vi "_STP.vi"(0 "System no.":i32=1 min=1 max=4 step=1, 2 "Affected axes?":string[](array[string]), 3 "All axes?":bool, 4 "Axis identifier?":bool=TRUE, 5 "error in":errorcluster) -> (19 "error out":errorcluster)   [LabVIEW 2018]
doc: "Stops motion of specified axes. To stop a referencing routine (REF, MNL, MPL) or fast scan routine (FSC, FSA etc.), or AutoZero procedure (ATZ), or wave generator run (WGO), use \"#24.vi\". STP sets error code 10, call \"ERR?.vi\" to reset error after STP has been called.\n\nValid for Analog systems, C-702, C-843, C-843.PM, C-844, C-848, C-865, C-866, C-867, C-880, E-516, E-517, E-712, E-725, E-753, E755, E-761, E-861, Mercury™ (but must be present for E-710 also). To support analog interfacing, VI must be present for E-816 also.\n\nAnalog: All axes = TRUE, Axis identifier = FALSE. STP does not set any error code.\nC-702: All axes = TRUE, Axis identifier = FALSE\nC-843: All axes = TRUE, Axis identifier = FALSE\nC-843.PM: All axes = TRUE, Axis identifier = FALSE\nC-844: All axes = TRUE, Axis identifier = FALSE\nC-848: All axes = TRUE, Axis identifier = FALSE\nC-865: All axes = TRUE, Axis identifier = FALSE\nC-866: All axes = TRUE, Axis identifier = FALSE\nC-867: All axes? = TRUE, Axis identifier? = FALSE\nC-880: All axes = TRUE, Axis identifier = FALSE \nE-516: If All axes = TRUE, then Axis identifier must be TRUE\nE-517: All axes? = TRUE, Axis identifier? = FALSE. STP.vi stops motion of all axes caused by move commands (MOV, MVR, GOH, SVA, SVR). Furthermore, it stops macros (MAC) and wave generator output (WGO).\nE-712, E-725, E-753: If All axes? = TRUE, then Axis identifier? can be FALSE. STP.vi stops motion of all axes caused by move commands (MOV, MVR, SVA, SVR), by the wave generator (WGO), by analog control input and autozero motion (ATZ).\nE-755: If All axes? = TRUE, then Axis identifier can be FALSE\nE-761: All axes = TRUE, Axis identifier = FALSE\nE-861: All axes? = TRUE, Axis identifier? = FALSE\nMercury: All axes = TRUE, Axis identifier = FALSE"
panel:
  # "Stops the motion of the specified axes.\n(To stop a referencing routine or firmware internal\nfast scan routines, or AutoZero procedure, or wave\ngenerator run, use \"#24.vi\")"
  # "If all axes: use"
  # "Stop"
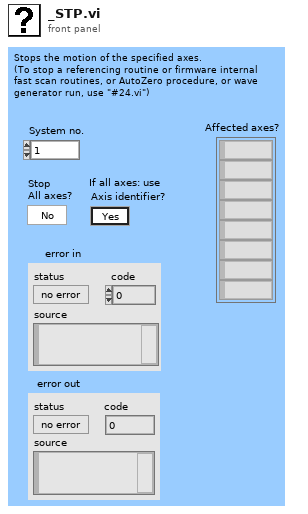
[diagram p1: front panel]
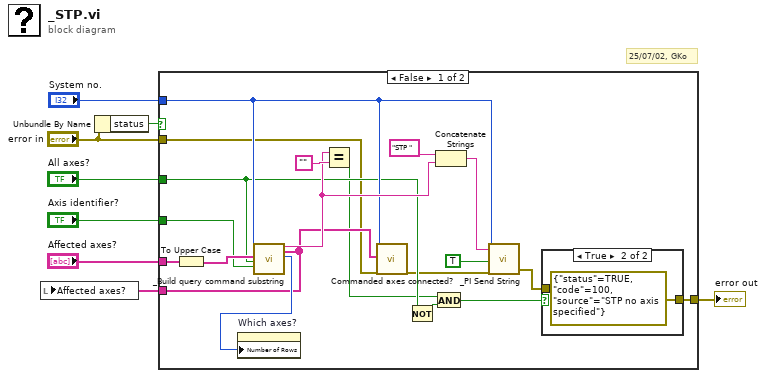
[diagram p0: block diagram]
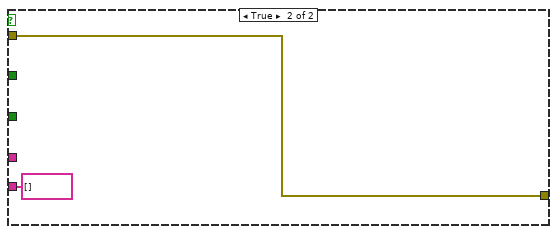
[diagram p3: hidden frame]
diagram:
  # "25/07/02, GKo"
  n1 = Unbundle By Name("error in") -> ("status"=w1:bool)
  n2 = case shown="False" w1 {
    tunnel: "Affected axes?" -> [w24 _]
    tunnel: [w21 w30] -> w7
    tunnel: "Axis identifier?" -> [w19 _]
    tunnel: "System no." -> [w16 _]
    tunnel: [w15 string[] [] ("Axes to query out")] -> w4
    tunnel: "All axes?" -> [w14 _]
    tunnel: "error in" -> [w9 w30]
    frame False {
      n3 = To Upper Case(1:w24) -> (0:w20:string[])
      n4 = call "_Build query command substring.vi"("System no."=w16, "Axes to query in"=w20, "Query\nAll axes?"=w14, "For all axes: use\nAxis identifier?"=w19) -> ("Command substring"=w18:string, "Axes to query out"=w15:string[], "Number of rows"=w17:u32)  [unwired: 13 in]
      n5 = property on="Which axes?" class="Arr (strict)"("Number of Rows"=w17) -> ()  [unwired: 2 in, 2 out]
      n6 = Equal?(x=w18, y="" ("x")) -> (x = y?=w13:bool)
      n7 = call "Commanded axes connected?.vi"("System no."=w16, "Commanded axes"=w15, "error in"=w9) -> ("error out"=w11:errorcluster)  [unwired: 15 in, 1 out]
      n8 = Not(x=w14) -> (.not. x?=w12:bool)
      n9 = And(x=w13, y=w12) -> (x .and. y?=w22:bool)
      n10 = Concatenate Strings("STP ", w18) -> (w25:string)
      n11 = call "_PI Send String.vi"("System no."=w16, "String to send"=w25, "Attach termination char.?"=TRUE ("Attach Linefeed?"), "error in"=w11) -> ("error out"=w10:errorcluster)  [unwired: 15 in]
      n12 = case shown="True" w22 {
        tunnel: [w28 errorcluster {"status"=TRUE, "code"=100, "source"="STP no axis specified"} ("error out")] -> w21
        tunnel: w10 -> [w28 _]
        frame False {
        }
        frame True {
        }
      }
    }
    frame True {
    }
  }
  "error out" <- w7
  n13 = local write "Affected axes?"(w4) -> ()
